vi "LS DAS File Save.vi"(0 "Raw Data":fxp<+/-,22,11>[](array[numeric]), 1 "ValidFifoRead":bool, 2 "Day In":i32, 3 "Count In":i32, 4 "Bank1 Filepath":path, 5 "Bank2 Filepath":path, 6 "Opens In":i32[](array[numeric]), 7 "Row Count In":i32, 8 "Bank2Slow":bool, 9 "LowRate":i32, 10 "Anomaly Filepath":path) -> (15 "Day Out":i32, 18 "Count Out":i32, 19 "Second File Count Out":i32)   [LabVIEW 2018]
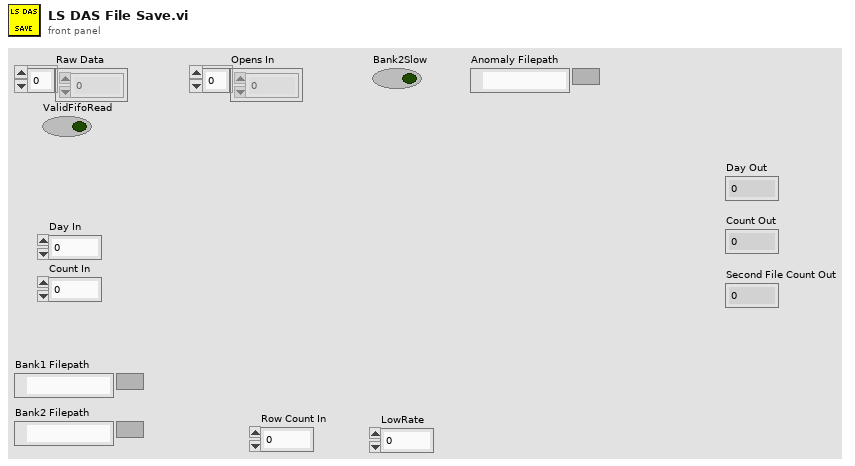
[diagram p1: front panel]
types:
  T1 = enum16{"open", "replace", "create", "open or create", "replace or create", "replace or create with confirmation"}
  T2 = typedef "LVDateTimeRec.ctl" = cluster{"fractional second":dbl, "second":i32, "minute":i32, "hour":i32, "day of month":i32, "month":i32, "year":i32, "day of week":i32, "day of year":i32, "DST":i32}
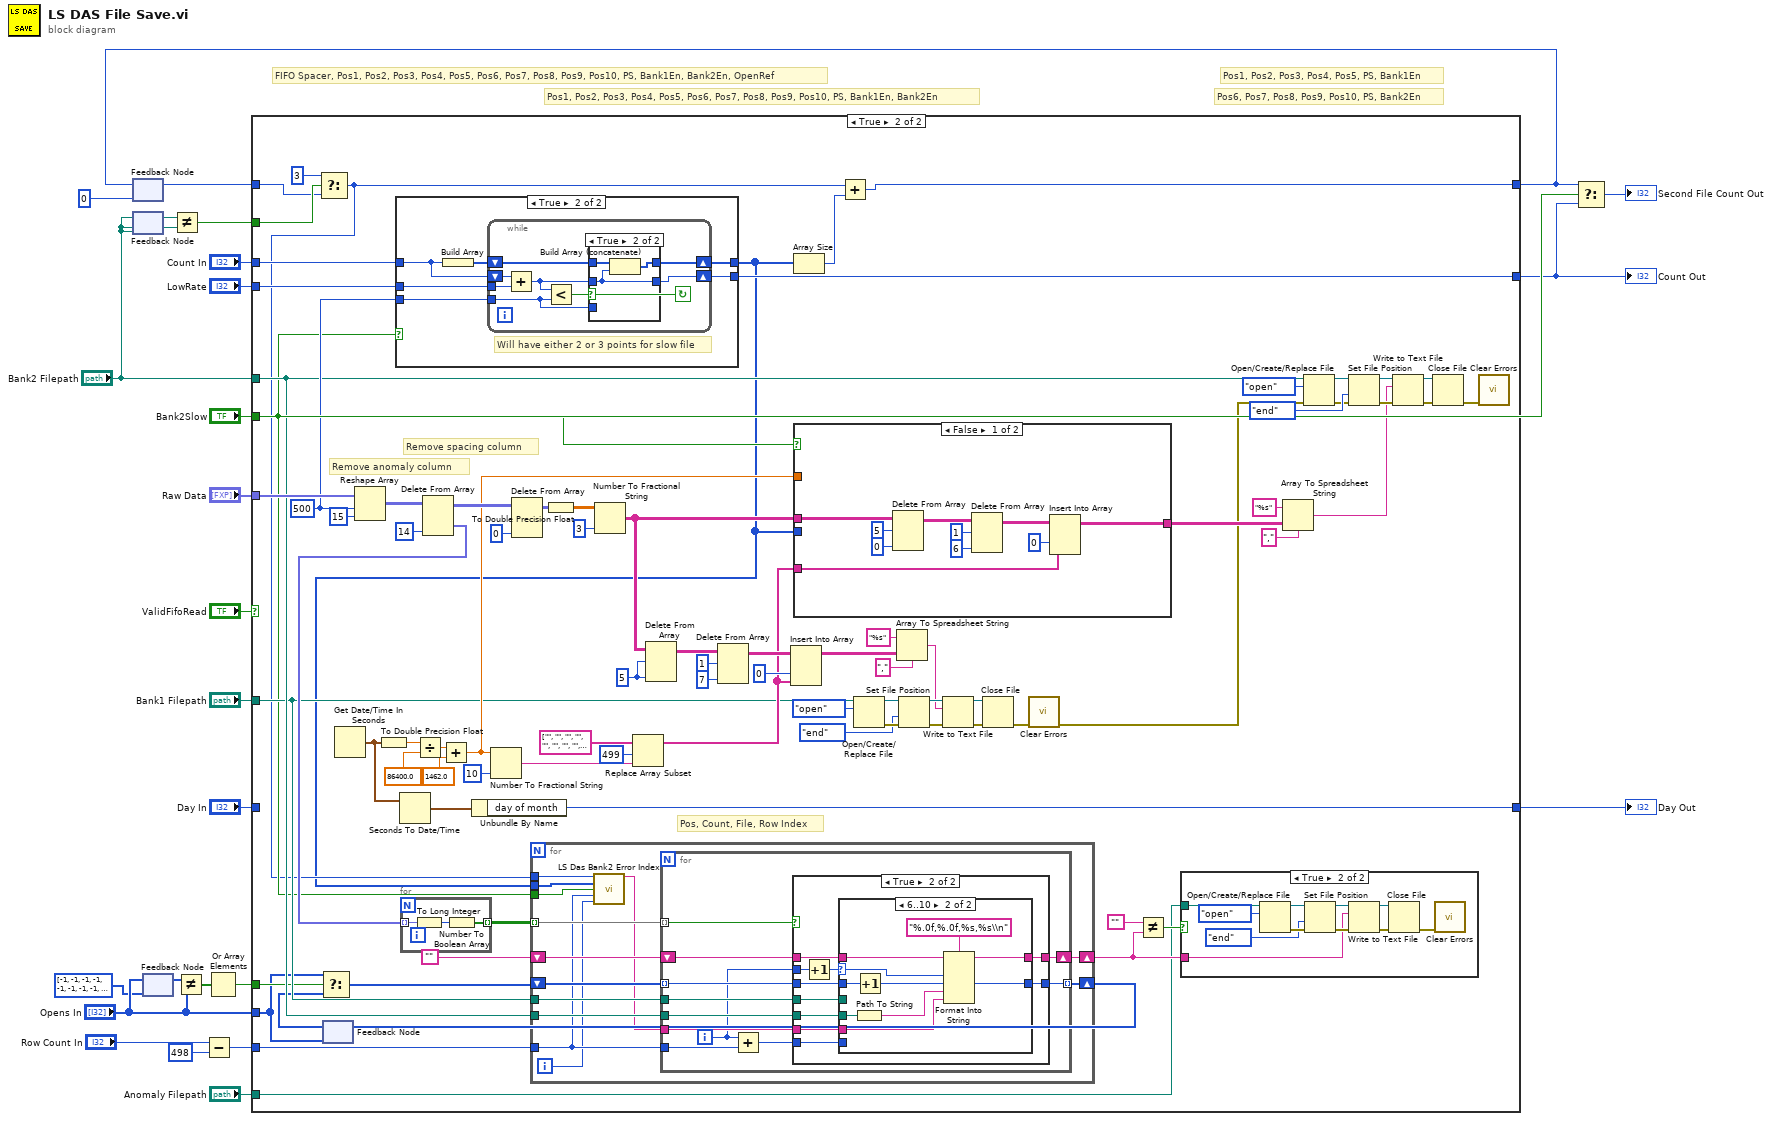
[diagram p0: block diagram]
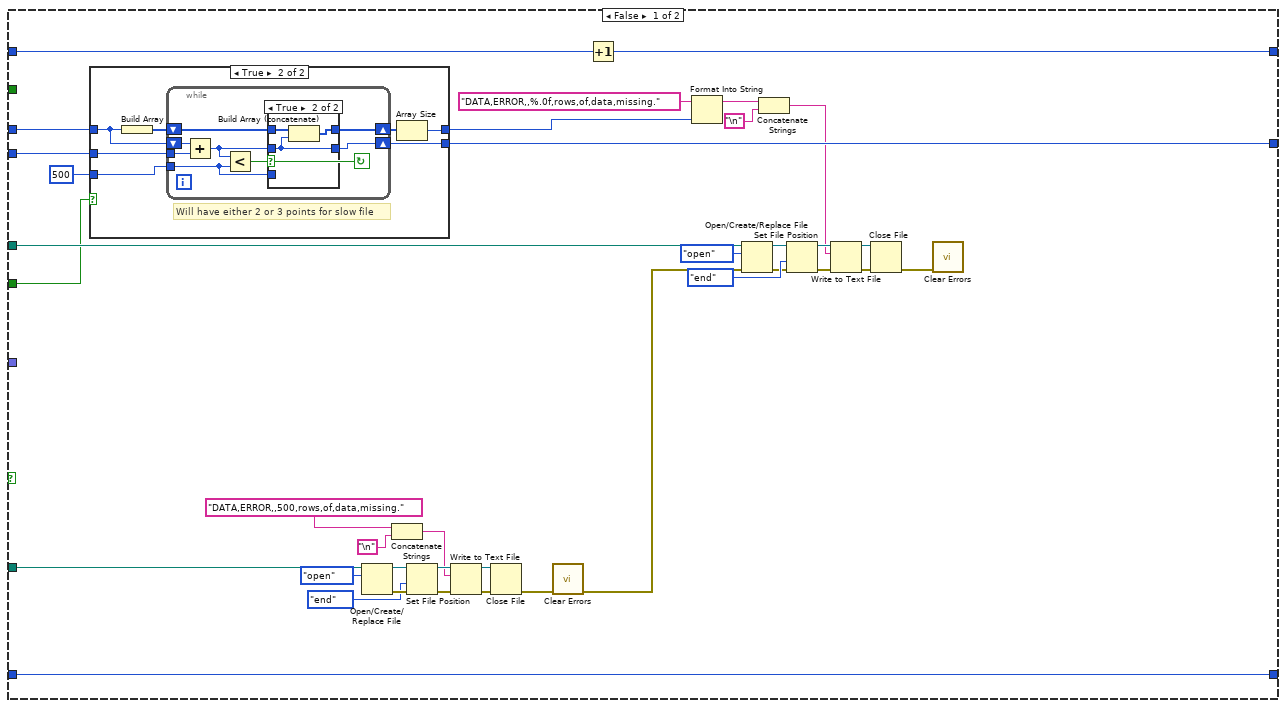
[diagram p2: hidden frame]
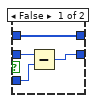
[diagram p4: hidden frame]
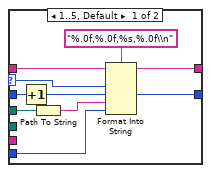
[diagram p7: hidden frame]
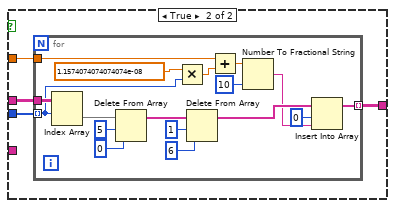
[diagram p8: hidden frame]
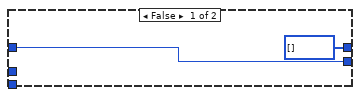
[diagram p9: hidden frame]
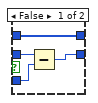
[diagram p10: hidden frame]
diagram:
  # "Pos1, Pos2, Pos3, Pos4, Pos5, Pos6, Pos7, Pos8, Pos9, Pos10, PS, Bank1En, Bank2En"
  # "Pos6, Pos7, Pos8, Pos9, Pos10, PS, Bank2En"
  # "Pos1, Pos2, Pos3, Pos4, Pos5, PS, Bank1En"
  # "FIFO Spacer, Pos1, Pos2, Pos3, Pos4, Pos5, Pos6, Pos7, Pos8, Pos9, Pos10, PS, Bank1En, Bank2En, OpenRef"
  n1 = feedback #1(0) -> (w14:i32)
  n2 = feedback-in #2("Bank2 Filepath") -> ()
  n3 = feedback #2("Bank2 Filepath") -> (w17:path)
  n4 = feedback-in #3("Opens In") -> ()
  n5 = feedback #3(i32[] [-1, -1, -1, -1, -1, -1, -1, -1, -1, -1] ("Opens In")) -> (w8:i32[])
  n6 = Not Equal?(x=w17, y="Bank2 Filepath") -> (x != y?=w16:bool)
  n7 = Not Equal?(x=w8, y="Opens In") -> (x != y?=w7:bool[])
  n8 = Subtract(x="Row Count In", y=498) -> (x-y=w2:i32)
  n9 = Or Array Elements(Boolean array=w7) -> (logical OR=w4:bool)
  n10 = case shown="True" "ValidFifoRead" {
    tunnel: [w58 w165] -> w25
    tunnel: "Raw Data" -> [_ w150]
    tunnel: "Day In" -> [w58 _]
    tunnel: "Bank1 Filepath" -> [w46 w106]
    tunnel: "Bank2 Filepath" -> [w36 w107]
    tunnel: "Count In" -> [w61 w135]
    tunnel: "LowRate" -> [w62 w136]
    tunnel: [w59 w133] -> w10
    tunnel: "Bank2Slow" -> [w28 w103]
    tunnel: "Opens In" -> [_ w88]
    tunnel: w2 -> [_ w108]
    tunnel: w16 -> [_ w102]
    tunnel: w14 -> [w27 w101]
    tunnel: [w26 w98] -> w11
    tunnel: "Anomaly Filepath" -> [_ w93]
    tunnel: w4 -> [_ w90]
    frame False {
      n11 = case shown="True" w28 {
        tunnel: w62 -> [_ w70]
        tunnel: w61 -> [w63 w69]
        tunnel: 500 ("dimension size") -> [w64 w68]
        tunnel: [w63 w67] -> w59
        tunnel: [w64 w65] -> w32
        frame False {
        }
        frame True {
          # "Will have either 2 or 3 points for slow file"
          n12 = Build Array(w69) -> (w71:i32[])
          n13 = while {
            shift-right: [w75] -> w66
            shift-left: w71 -> [w77]
            tunnel: w70 -> [w78]
            shift-right: [w74] -> w67
            shift-left: w69 -> [w79]
            tunnel: w68 -> [w73]
            stop <- w72 continue-if-true
            n14 = Add(x=w79, y=w78) -> (x+y=w76:i32)
            n15 = Less?(x=w76, y=w73) -> (x < y?=w72:bool)
            n16 = case shown="True" w72 {
              tunnel: w77 -> [w83 w86]
              tunnel: w76 -> [w82 w84]
              tunnel: [w83 w85] -> w75
              tunnel: [w80 w84] -> w74
              tunnel: w73 -> [w81 _]
              frame False {
                n17 = Subtract(x=w82, y=w81) -> (x-y=w80:i32)
              }
              frame True {
                n18 = Build Array (concatenate)(w86, w84) -> (w85:i32[])
              }
            }
          }
          n19 = Array Size(array=w66) -> (size(s)=w65:i32)
        }
      }
      n20 = Open/Create/Replace File(file path (use dialog)=w46, operation (0:open)=T1."open") -> (refnum out=w51:refnum<file>, error out=w50:errorcluster)  [unwired: 4 in, 1 out]
      n21 = Concatenate Strings("DATA,ERROR,,500,rows,of,data,missing." ("string"), "\n") -> (w29:string)
      n22 = Set File Position(refnum=w51, from (0:start)=enum16{"start", "end", "current"}."end", error in=w50) -> (refnum out=w48:refnum<file>, error out=w47:errorcluster)  [unwired: 1 in]
      n23 = Write to Text File(file (use dialog)=w48, text=w29, error in=w47) -> (refnum out=w54:refnum<file>, error out=w55:errorcluster)  [unwired: 1 in, 1 out]
      n24 = Close File(refnum=w54, error in=w55) -> (error out=w53:errorcluster)  [unwired: 1 out]
      n25 = call <vilib>:"Clear Errors.vi"("error in (no error)"=w53) -> ("error out"=w35:errorcluster)  [unwired: 5 in, 1 out]
      n26 = Increment(x=w27) -> (x+1=w26:i32)
      n27 = Format Into String(initial string="DATA,ERROR,,%.0f,rows,of,data,missing." ("input string"), w32) -> (resulting string=w31:string)  [unwired: 2 in, 1 out]
      n28 = Open/Create/Replace File(file path (use dialog)=w36, error in=w35, operation (0:open)=T1."open") -> (refnum out=w41:refnum<file>, error out=w42:errorcluster)  [unwired: 3 in, 1 out]
      n29 = Concatenate Strings(w31, "\n") -> (w30:string)
      n30 = Set File Position(refnum=w41, from (0:start)=enum16{"start", "end", "current"}."end", error in=w42) -> (refnum out=w44:refnum<file>, error out=w45:errorcluster)  [unwired: 1 in]
      n31 = Write to Text File(file (use dialog)=w44, text=w30, error in=w45) -> (refnum out=w38:refnum<file>, error out=w37:errorcluster)  [unwired: 1 in, 1 out]
      n32 = Close File(refnum=w38, error in=w37) -> (error out=w39:errorcluster)  [unwired: 1 out]
      n33 = call <vilib>:"Clear Errors.vi"("error in (no error)"=w39) -> ()  [unwired: 5 in, 2 out]
    }
    frame True {
      w117 = 5 ("disabled index (col)")
      w134 = 500 ("dimension size")
      # "Pos, Count, File, Row Index"
      # "Remove spacing column"
      # "Remove anomaly column"
      n34 = Select(t=3, s=w102, f=w101) -> (s? t:f=w97:i32)
      n35 = feedback #4(w88) -> (w89:i32[])
      n36 = Select(t=w88, s=w90, f=w89) -> (s? t:f=w87:i32[])
      n37 = Get Date/Time In Seconds() -> (seconds since 1Jan1904=w155:timestamp)
      n38 = Reshape Array(w150, w134, 15 ("dimension size")) -> (w152:fxp<+/-,22,11>[][])
      n39 = To Double Precision Float(number=w155) -> (double precision float=w157:dbl)
      n40 = case shown="True" w103 {
        tunnel: w136 -> [_ w275]
        tunnel: w135 -> [w270 w274]
        tunnel: w134 -> [_ w273]
        tunnel: [w270 w272] -> w133
        tunnel: [i32[] [] w271] -> w96
        frame False {
        }
        frame True {
          # "Will have either 2 or 3 points for slow file"
          n41 = Build Array(w274) -> (w276:i32[])
          n42 = while {
            shift-right: [w280] -> w271
            shift-left: w276 -> [w282]
            tunnel: w275 -> [w283]
            shift-right: [w279] -> w272
            shift-left: w274 -> [w284]
            tunnel: w273 -> [w278]
            stop <- w277 continue-if-true
            n43 = Add(x=w284, y=w283) -> (x+y=w281:i32)
            n44 = Less?(x=w281, y=w278) -> (x < y?=w277:bool)
            n45 = case shown="True" w277 {
              tunnel: w282 -> [w288 w291]
              tunnel: w281 -> [w287 w289]
              tunnel: [w288 w290] -> w280
              tunnel: [w285 w289] -> w279
              tunnel: w278 -> [w286 _]
              frame False {
                n46 = Subtract(x=w287, y=w286) -> (x-y=w285:i32)
              }
              frame True {
                n47 = Build Array (concatenate)(w291, w289) -> (w290:i32[])
              }
            }
          }
        }
      }
      n48 = Seconds To Date/Time(time stamp (now)=w155) -> (date time rec=w154:T2)  [unwired: 1 in]
      n49 = Divide(x=w157, y=86400.0) -> (x/y=w159:dbl)
      n50 = Delete From Array(array=w152, index (col)=14 ("disabled index (col)")) -> (deleted portion=w109:fxp<+/-,22,11>[], array with subset deleted=w166:fxp<+/-,22,11>[][])  [unwired: 2 in]
      n51 = for {
        tunnel: w109 -> [w235] mode=indexing
        tunnel: [w236] -> w92 mode=indexing
        n52 = To Long Integer(number=w235) -> (32bit integer=w237:i32)
        n53 = Number To Boolean Array(number=w237) -> (Boolean array=w236:bool[])
      }
      n54 = Add(x=w159, y=1462.0) -> (x+y=w119:dbl)
      n55 = Unbundle By Name(w154) -> ("day of month"=w165:i32)
      n56 = Number To Fractional String(number=w119, precision (6)=i16 10) -> (F-format string=w156:string)  [unwired: 2 in]
      n57 = Delete From Array(array=w166, index (col)=0 ("disabled index (col)")) -> (array with subset deleted=w168:fxp<+/-,22,11>[][])  [unwired: 2 in, 1 out]
      n58 = for {
        tunnel: w92 -> [w193] mode=indexing
        tunnel: w108 -> [w182]
        shift-right: [w192] -> w91
        shift-left: w87 -> [w191]
        tunnel: w107 -> [w190]
        tunnel: w106 -> [w189]
        shift-right: [w187] -> w94
        shift-left: "" -> [w188]
        tunnel: w103 -> [w184]
        tunnel: w97 -> [w186]
        tunnel: w96 -> [w185]
        i -> [w181]
        n59 = call "LS Das Bank2 Error Index.vi"("RowCountSlow"=w186, "SlowRecordIndexes"=w185, "Bank2SlowRecord"=w184, "RowCountStandard"=w182, "ErrorIndex"=w181) -> ("Bank2ErrorIndex"=w183:string)  [unwired: 10 in]
        n60 = for {
          tunnel: w193 -> [w204] mode=indexing
          tunnel: w191 -> [w203] mode=indexing
          tunnel: [w202] -> w192 mode=indexing
          tunnel: w190 -> [w201]
          tunnel: w189 -> [w200]
          shift-right: [w198] -> w187
          shift-left: w188 -> [w199]
          tunnel: w182 -> [w196]
          tunnel: w183 -> [w195]
          i -> [w194]
          n61 = Add(x=w194, y=w196) -> (x+y=w197:i32)
          n62 = case shown="True" w204 {
            tunnel: w194 -> [_ w210]
            tunnel: w203 -> [w205 w216]
            tunnel: [w205 w215] -> w202
            tunnel: w201 -> [_ w214]
            tunnel: w200 -> [_ w213]
            tunnel: w199 -> [w206 w212]
            tunnel: [w206 w211] -> w198
            tunnel: w197 -> [_ w208]
            tunnel: w195 -> [_ w207]
            frame False {
            }
            frame True {
              n63 = Increment(x=w210) -> (x+1=w209:i32)
              n64 = case shown="6..10" w209 {
                selector: w209 -> [w220 w229]
                tunnel: w216 -> [w224 w233]
                tunnel: [w223 w232] -> w215
                tunnel: w214 -> [_ w227]
                tunnel: w213 -> [w217 _]
                tunnel: w212 -> [w222 w231]
                tunnel: [w221 w230] -> w211
                tunnel: w208 -> [w218 _]
                tunnel: w207 -> [_ w226]
                frame 1..5, Default {
                  n65 = Increment(x=w224) -> (x+1=w223:i32)
                  n66 = Path To String(path=w217) -> (string=w219:string)
                  n67 = Format Into String(format string="%.0f,%.0f,%s,%.0f\\n" ("initial string"), initial string=w222, w220, w223, w219, w218) -> (resulting string=w221:string)  [unwired: 1 in, 1 out]
                }
                frame 6..10 {
                  n68 = Path To String(path=w227) -> (string=w228:string)
                  n69 = Increment(x=w233) -> (x+1=w232:i32)
                  n70 = Format Into String(format string="%.0f,%.0f,%s,%s\\n" ("initial string"), initial string=w231, w229, w232, w228, w226) -> (resulting string=w230:string)  [unwired: 1 in, 1 out]
                }
              }
            }
          }
        }
      }
      n71 = feedback-in #4(w91) -> ()
      n72 = To Double Precision Float(number=w168) -> (double precision float=w169:dbl[][])
      n73 = Number To Fractional String(number=w169, precision (6)=i16 3) -> (F-format string=w112:string[][])  [unwired: 2 in]
      n74 = Replace Array Subset(array=string[] ["", "", "", "", "", "", "", "", "", "", "", "", "", "", "", "", "", "", "", "", "", "", "", "", "", "", "", "", "", "", "", "", "", "", "", "", "", "", "", "", "", "", "", "", "", "", "", "", "", "", "", "", "", "", "", "", "", "", "", "", "", "", "", "", "", "", "", "", "", "", "", "", "", "", "", "", "", "", "", "", "", "", "", "", "", "", "", "", "", "", "", "", "", "", "", "", "", "", "", "", "", "", "", "", "", "", "", "", "", "", "", "", "", "", "", "", "", "", "", "", "", "", "", "", "", "", "", "", "", "", "", "", "", "", "", "", "", "", "", "", "", "", "", "", "", "", "", "", "", "", "", "", "", "", "", "", "", "", "", "", "", "", "", "", "", "", "", "", "", "", "", "", "", "", "", "", "", "", "", "", "", "", "", "", "", "", "", "", "", "", "", "", "", "", "", "", "", "", "", "", "", "", "", "", "", "", "", "", "", "", "", "", "", "", "", "", "", "", "", "", "", "", "", "", "", "", "", "", "", "", "", "", "", "", "", "", "", "", "", "", "", "", "", "", "", "", "", "", "", "", "", "", "", "", "", "", "", "", "", "", "", "", "", "", "", "", "", "", "", "", "", "", "", "", "", "", "", "", "", "", "", "", "", "", "", "", "", "", "", "", "", "", "", "", "", "", "", "", "", "", "", "", "", "", "", "", "", "", "", "", "", "", "", "", "", "", "", "", "", "", "", "", "", "", "", "", "", "", "", "", "", "", "", "", "", "", "", "", "", "", "", "", "", "", "", "", "", "", "", "", "", "", "", "", "", "", "", "", "", "", "", "", "", "", "", "", "", "", "", "", "", "", "", "", "", "", "", "", "", "", "", "", "", "", "", "", "", "", "", "", "", "", "", "", "", "", "", "", "", "", "", "", "", "", "", "", "", "", "", "", "", "", "", "", "", "", "", "", "", "", "", "", "", "", "", "", "", "", "", "", "", "", "", "", "", "", "", "", "", "", "", "", "", "", "", "", "", "", "", "", "", "", "", "", "", "", "", "", "", "", "", "", "", "", "", "", "", "", "", "", "", "", "", "", "", "", "", "", "", "", "", "", "", "", "", "", "", "", "", "", "", "", "", "", "", "", "", "", "", ""], new element=w156, index=499) -> (w110:string[])
      n75 = Delete From Array(array=w112, length=w117, index (col)=w117) -> (array with subset deleted=w116:string[][])  [unwired: 1 in, 1 out]
      n76 = Delete From Array(array=w116, length=1, index (col)=7 ("disabled index (col)")) -> (array with subset deleted=w113:string[][])  [unwired: 1 in, 1 out]
      n77 = Insert Into Array(array=w113, index (col)=0 ("disabled index (col)"), new element=w110) -> (w111:string[][])  [unwired: 1 in]
      n78 = Array Size(array=w96) -> (size(s)=w99:i32)
      n79 = case shown="False" w103 {
        tunnel: w112 -> [w247 w251]
        tunnel: [w241 w250] -> w121
        tunnel: w119 -> [_ w249]
        tunnel: w96 -> [_ w248]
        tunnel: w110 -> [w239 _]
        frame False {
          n80 = Delete From Array(array=w247, length=5, index (col)=0 ("disabled index (col)")) -> (array with subset deleted=w244:string[][])  [unwired: 1 in, 1 out]
          n81 = Delete From Array(array=w244, length=1, index (col)=6 ("disabled index (col)")) -> (array with subset deleted=w242:string[][])  [unwired: 1 in, 1 out]
          n82 = Insert Into Array(array=w242, index (col)=0 ("disabled index (col)"), new element=w239) -> (w241:string[][])  [unwired: 1 in]
        }
        frame True {
          n83 = for {
            tunnel: w248 -> [w264] mode=indexing
            tunnel: w251 -> [w268]
            tunnel: w249 -> [w265]
            tunnel: [w254] -> w250 mode=indexing
            n84 = Index Array(array=w268, index (row)=w264) -> (element=w258:string[])  [unwired: 1 in]
            n85 = Delete From Array(array=w258, length=5, index=0) -> (array with subset deleted=w257:string[])  [unwired: 1 out]
            n86 = Multiply(x=1.1574074074074074e-08, y=w264) -> (x*y=w263:dbl)
            n87 = Delete From Array(array=w257, length=1 ("index"), index=6 ("length")) -> (array with subset deleted=w256:string[])  [unwired: 1 out]
            n88 = Add(x=w265, y=w263) -> (x+y=w262:dbl)
            n89 = Number To Fractional String(number=w262, precision (6)=i16 10) -> (F-format string=w255:string)  [unwired: 2 in]
            n90 = Insert Into Array(array=w256, index=0, new element=w255) -> (w254:string[])
          }
        }
      }
      n91 = Add(x=w97, y=w99) -> (x+y=w98:i32)
      n92 = Open/Create/Replace File(file path (use dialog)=w106, operation (0:open)=T1."open") -> (refnum out=w144:refnum<file>, error out=w143:errorcluster)  [unwired: 4 in, 1 out]
      n93 = Array To Spreadsheet String(delimiter (Tab)=",", array=w111, 3:"%s" ("format string")) -> (spreadsheet string=w137:string)
      n94 = Set File Position(refnum=w144, from (0:start)=enum16{"start", "end", "current"}."end", error in=w143) -> (refnum out=w141:refnum<file>, error out=w140:errorcluster)  [unwired: 1 in]
      n95 = Write to Text File(file (use dialog)=w141, text=w137, error in=w140) -> (refnum out=w147:refnum<file>, error out=w148:errorcluster)  [unwired: 1 in, 1 out]
      n96 = Close File(refnum=w147, error in=w148) -> (error out=w146:errorcluster)  [unwired: 1 out]
      n97 = call <vilib>:"Clear Errors.vi"("error in (no error)"=w146) -> ("error out"=w118:errorcluster)  [unwired: 5 in, 1 out]
      n98 = Not Equal?(x="", y=w94) -> (x != y?=w95:bool)
      n99 = case shown="True" w95 {
        tunnel: w94 -> [_ w171]
        tunnel: w93 -> [_ w170]
        frame False {
        }
        frame True {
          n100 = Open/Create/Replace File(file path (use dialog)=w170, operation (0:open)=T1."open") -> (refnum out=w176:refnum<file>, error out=w175:errorcluster)  [unwired: 4 in, 1 out]
          n101 = Set File Position(refnum=w176, from (0:start)=enum16{"start", "end", "current"}."end", error in=w175) -> (refnum out=w173:refnum<file>, error out=w172:errorcluster)  [unwired: 1 in]
          n102 = Write to Text File(file (use dialog)=w173, text=w171, error in=w172) -> (refnum out=w179:refnum<file>, error out=w180:errorcluster)  [unwired: 1 in, 1 out]
          n103 = Close File(refnum=w179, error in=w180) -> (error out=w178:errorcluster)  [unwired: 1 out]
          n104 = call <vilib>:"Clear Errors.vi"("error in (no error)"=w178) -> ()  [unwired: 5 in, 2 out]
        }
      }
      n105 = Array To Spreadsheet String(delimiter (Tab)=",", array=w121, 3:"%s" ("format string")) -> (spreadsheet string=w120:string)
      n106 = Open/Create/Replace File(file path (use dialog)=w107, error in=w118, operation (0:open)=T1."open") -> (refnum out=w128:refnum<file>, error out=w129:errorcluster)  [unwired: 3 in, 1 out]
      n107 = Set File Position(refnum=w128, from (0:start)=enum16{"start", "end", "current"}."end", error in=w129) -> (refnum out=w131:refnum<file>, error out=w132:errorcluster)  [unwired: 1 in]
      n108 = Write to Text File(file (use dialog)=w131, text=w120, error in=w132) -> (refnum out=w125:refnum<file>, error out=w124:errorcluster)  [unwired: 1 in, 1 out]
      n109 = Close File(refnum=w125, error in=w124) -> (error out=w126:errorcluster)  [unwired: 1 out]
      n110 = call <vilib>:"Clear Errors.vi"("error in (no error)"=w126) -> ()  [unwired: 5 in, 2 out]
    }
  }
  "Day Out" <- w25
  "Count Out" <- w10
  n111 = feedback-in #1(w11) -> ()
  n112 = Select(t=w11, s="Bank2Slow", f=w10) -> (s? t:f=→"Second File Count Out":i32)
